vi "Save Config INI to File.vi"(7 "File Type":string(combo)=".ini", 8 "Error In":errorcluster, 10 "reference":refnum<vi>, 11 "Path In":path) -> (0 "Error Out":errorcluster, 3 "Path Out":path)   [LabVIEW 2015]
uses:
  <vilib>/Utility/config.llb/Write Key (String).vi
  <vilib>/Utility/config.llb/NI_LVConfig.lvlib
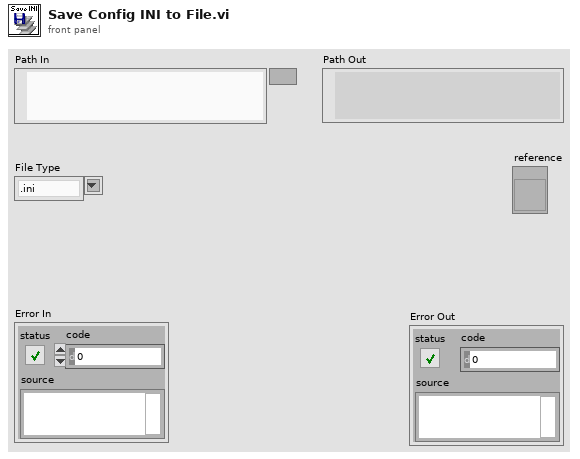
[diagram p1: front panel]
types:
  T1 = typedef "NI_LVConfig.lvlib/Config Data RefNum.ctl" = refnum<k1>
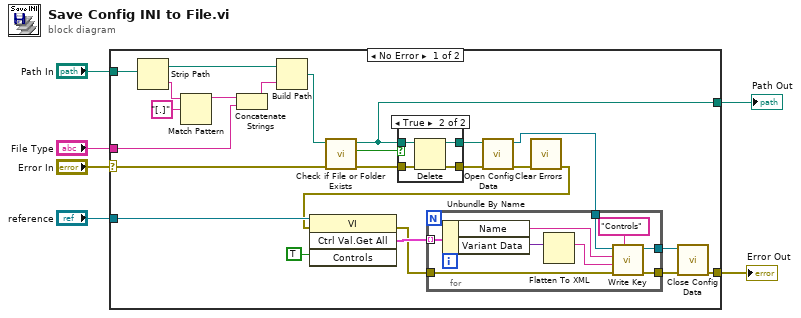
[diagram p0: block diagram]
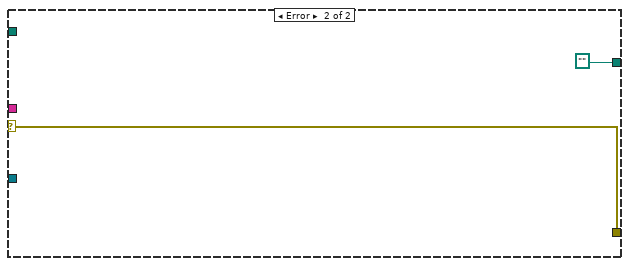
[diagram p3: hidden frame]
diagram:
  n1 = case shown="No Error" "Error In" {
    selector: "Error In" -> [w19 w47]
    tunnel: [w13 w47] -> w1
    tunnel: [w11 path ""] -> w6
    tunnel: "Path In" -> [w12 _]
    tunnel: "File Type" -> [w10 _]
    tunnel: "reference" -> [w9 _]
    frame No Error {
      n2 = Strip Path(path=w12) -> (stripped path=w29:path, name=w26:string)
      n3 = Match Pattern(string=w26, regular expression="[.]" ("search string")) -> (before substring=w27:string)  [unwired: 1 in, 3 out]
      n4 = Concatenate Strings(w27, w10) -> (w25:string)
      n5 = Build Path(base path=w29, name or relative path=w25) -> (appended path=w20:path)
      n6 = call <vilib>:"Check if File or Folder Exists.vi"("error in (no error)"=w19, "path"=w20) -> ("error out"=w23:errorcluster, "file or folder exists?"=w24:bool, "dup path"=w11:path)  [unwired: 7 in]
      n7 = case shown="True" w24 {
        tunnel: w23 -> [w40 w45]
        tunnel: w11 -> [w41 w44]
        tunnel: [w41 w43] -> w22
        tunnel: [w40 w42] -> w21
        frame False {
        }
        frame True {
          n8 = Delete(path (use dialog)=w44, error in=w45) -> (deleted path=w43:path, error out=w42:errorcluster)  [unwired: 3 in, 1 out]
        }
      }
      n9 = call <vilib>:"Open Config Data.vi"("error in (no error)"=w21, "configuration file path"=w22) -> ("error out"=w8:errorcluster, "refnum"=w17:T1)  [unwired: 1 in, 7 out]
      n10 = call <vilib>:"Clear Errors.vi"("error in (no error)"=w8) -> ("error out"=w7:errorcluster)  [unwired: 5 in, 1 out]
      n11 = invoke class="VI" method="Ctrl Val.Get All"(reference=w9, error in=w7, "Controls"=TRUE) -> (error out=w16:errorcluster, "Get All Control Values Variant"=w18:cluster{"Name":string, "Variant Data":variant}[])  [unwired: 1 in, 2 out]
      n12 = for {
        tunnel: w18 -> [w39] mode=indexing
        tunnel: w17 -> [w36]
        tunnel: w16 -> [w35]
        tunnel: [w32] -> w15
        tunnel: [w31] -> w14
        n13 = Unbundle By Name(w39) -> ("Name"=w34:string, "Variant Data"=w38:variant)
        n14 = Flatten To XML(anything=w38) -> (xml string=w33:string)
        n15 = call-poly <vilib>:"Write Key.vi"("section"="Controls", "error in (no error)"=w35, "value"=w33, "key"=w34, "refnum"=w36) -> ("error out"=w31:errorcluster, "refnum out"=w32:T1)  [unwired: 4 in, 1 out]
      }
      n16 = call <vilib>:"Close Config Data.vi"("error in (no error)"=w14, "refnum"=w15) -> ("error out"=w13:errorcluster)  [unwired: 1 in, 8 out]
    }
    frame Error {
      (unwired) ""
    }
  }
  "Path Out" <- w6
  "Error Out" <- w1
